vi "Experiment RT Servo.vi"(10 "Experiment Inputs":T2={"Duration"=5.0, "Initialisation Time"=1.0, "Sample Rate (Hz)"=200.0, "signal_type"=enum."Square", "Frequency"=0.5, "Amplitude"=1.0, "Offset"=2.5, "Velocity_feedback_gain"=0.1, "Feedforward_gain"=0.8, "LED_GAIN"=0.0, "LED_OFFSET"=0.0, "initial_condition"=0.0}) -> (0 "Error Out":errorcluster, 2 "Experiment Outputs":T4)   [LabVIEW 2016]
uses:
  Controls/Experiment Inputs.ctl
  Controls/Signal Type.ctl
  Controls/Experiment Outputs.ctl
  RT - Controls/Experiment RT State.ctl
  RT - Controls/Machine Data - RT.ctl
  <vilib>/Platform/TimedLoop/XDataNode/timing_clust.ctl
  <vilib>/Platform/TimedLoop/XDataNode/nitl_modes.ctl
  <vilib>/Platform/TimedLoop/XDataNode/wakeup.ctl
  Controller/Controller Values.ctl
  Pauseable Timer/Timer Mode.ctl
  <vilib>/Platform/TimedLoop/XDataNode/XDataNode.xnode
  <vilib>/ptbypt/NI_PtbyPt.lvlib
  <vilib>/Platform/TimedLoop/XDataNode/XDNodeRunTimeDep.lvlib
panel:
  out "Experiment RT State":T1
  in  "Error In":errorcluster
  out "Experiment Inputs Out":T2={"Duration"=5.0, "Initialisation Time"=1.0, "Sample Rate (Hz)"=200.0, "signal_type"=enum."Square", "Frequency"=0.5, "Amplitude"=1.0, "Offset"=2.5, "Velocity_feedback_gain"=0.1, "Feedforward_gain"=0.8, "LED_GAIN"=0.0, "LED_OFFSET"=0.0, "initial_condition"=0.0}
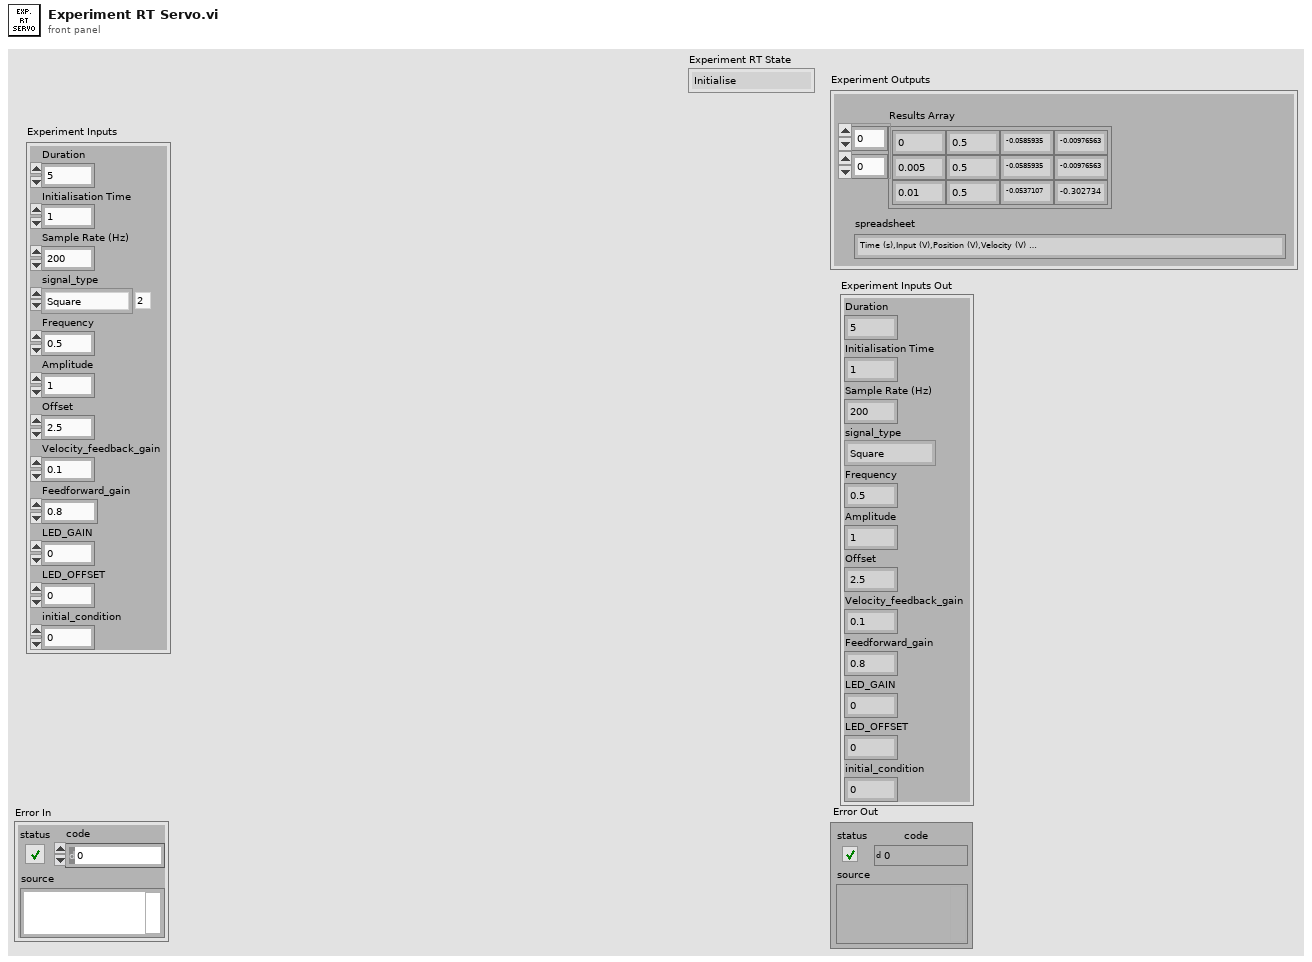
[diagram p1: front panel]
types:
  T1 = typedef "Experiment RT State.ctl" = enum16{"Initialise", "Wait Initialise", "Experiment", "End Experiment", "Quit"}
  T2 = typedef "Experiment Inputs.ctl" = cluster{"Duration":dbl, "Initialisation Time":dbl, "Sample Rate (Hz)":dbl, "signal_type":T3, "Frequency":dbl, "Amplitude":dbl, "Offset":dbl, "Velocity_feedback_gain":dbl, "Feedforward_gain":dbl, "LED_GAIN":dbl, "LED_OFFSET":dbl, "initial_condition":dbl}
  T3 = typedef "Signal Type.ctl" = enum16{"Sine", "Cosine", "Square", "Step"}
  T4 = typedef "Experiment Outputs.ctl" = cluster{"Results Array":dbl[][], "spreadsheet":string}
  T5 = typedef "Machine Data - RT.ctl" = cluster{"Results Array":dbl[][], "Motor Output":dbl, "LED Output":dbl, "Sample Index":u32, "Req. Samples":u32}
  T6 = typedef "XDNodeRunTimeDep.lvlib/timing_clust.ctl" = cluster{"Expected End [f-1]":u64, "Actual End [f-1]":u64, "Finished Late? [f-1]":bool, "Expected End [i-1]":u64, "Actual End [i-1]":u64, "Finished Late? [i-1]":bool, "Expected Start [i]":u64, "Actual Start [i]":u64, "Expected Start [f]":u64, "Actual Start [f]":u64, "Source Name":string, "Structure Name":string, "Period":i64, "Deadline":i64, "Offset":i64, "Start":i64, "Priority":i32, "Timeout":i32, "Mode":T7, "Wakeup Reason":T8, "Error":errorcluster, "Source Type":string, "Secondary Source Type":string, "Global End Time":u64, "Global Start Time":u64, "Frame Duration":u64, "Iteration Duration":u64, "Assigned CPU":i32, "I/O Scan Engine Mode":u32}
  T7 = typedef "XDNodeRunTimeDep.lvlib/nitl_modes.ctl" = enum32{"No Change", "Process missed periods, maintain original phase", "Discard missed periods, maintain original phase", "Process missed periods, ignore original phase", "Discard missed periods, ignore original phase"}
  T8 = typedef "XDNodeRunTimeDep.lvlib/wakeup.ctl" = enum32{"Normal", "Aborted", "Asynchronous wakeup", "Timing source error", "Timed loop error", "Timeout"}
  T9 = typedef "Controller Values.ctl" = cluster{"Ka":dbl, "Kt":dbl, "Offset":dbl}
  T10 = typedef "Timer Mode.ctl" = enum16{"Initialise", "Read", "Pause"}
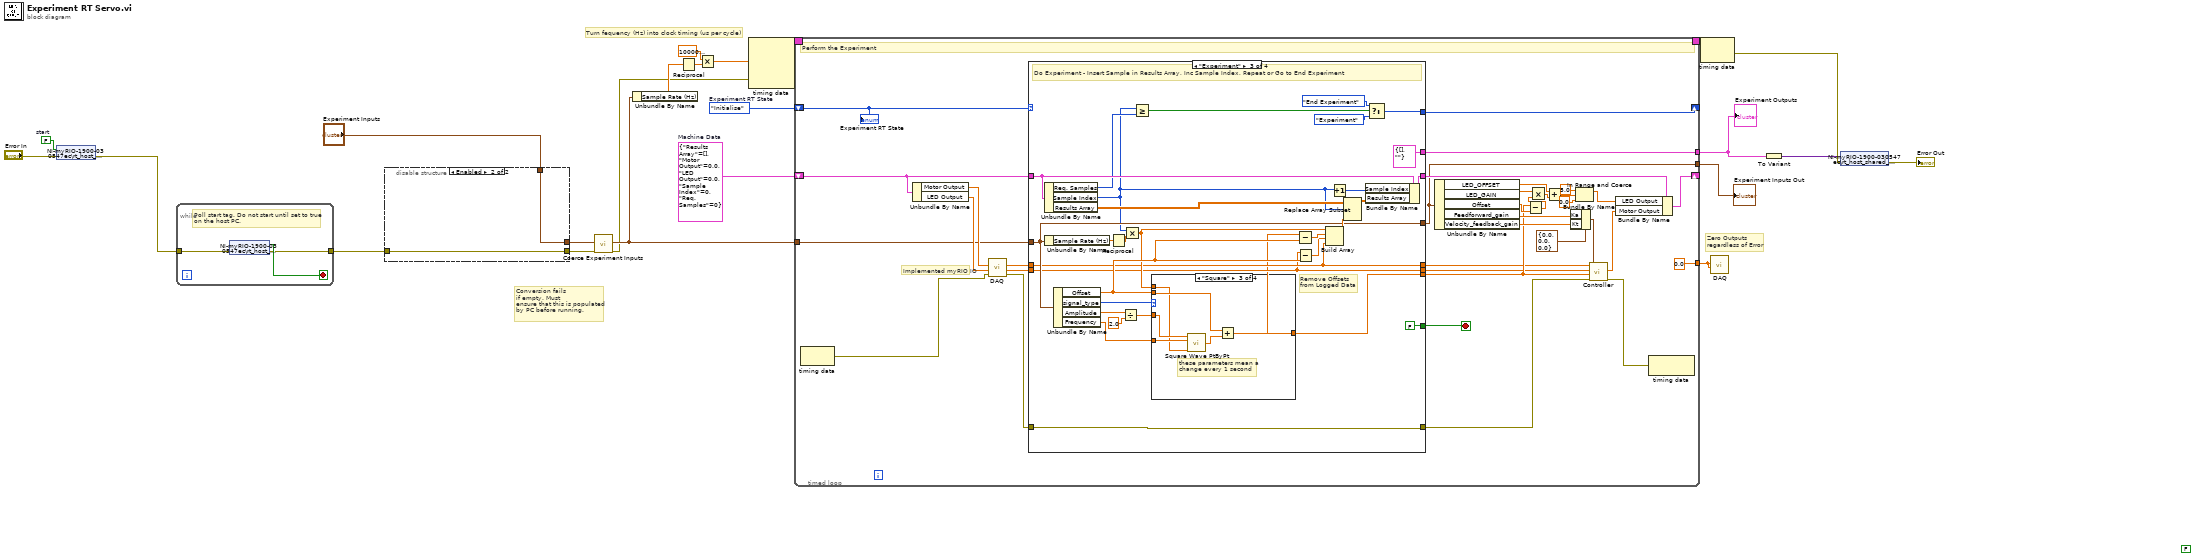
[diagram p0: block diagram]
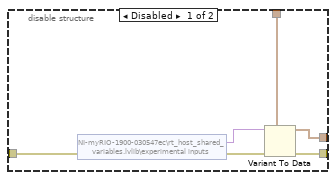
[diagram p2: hidden frame]
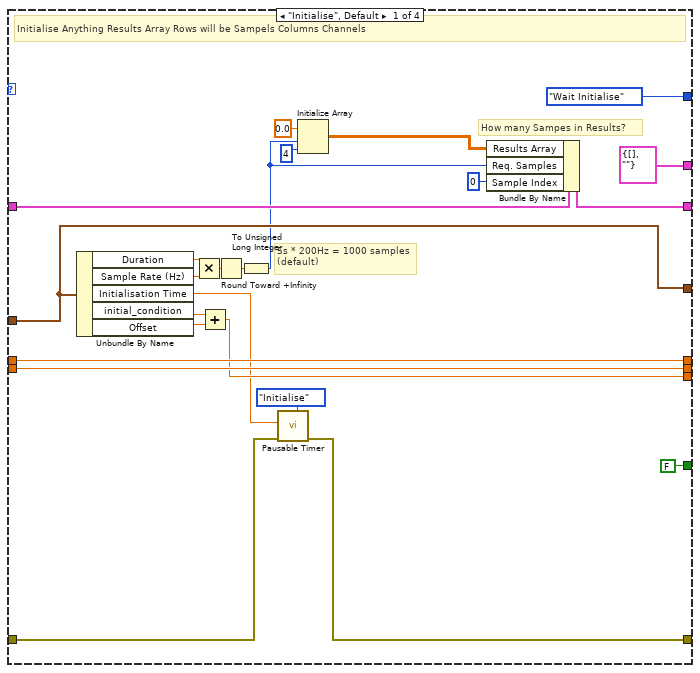
[diagram p3: hidden frame]
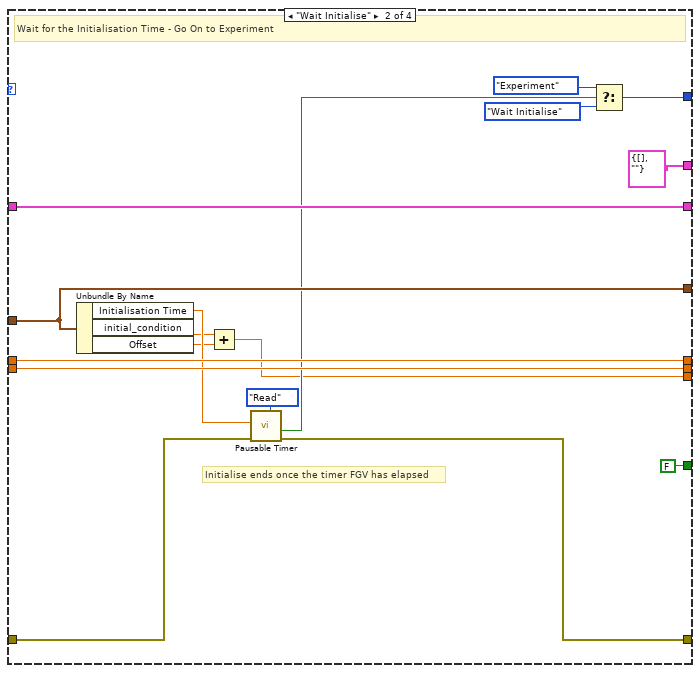
[diagram p4: hidden frame]
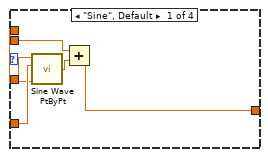
[diagram p5: hidden frame]
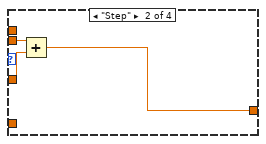
[diagram p6: hidden frame]
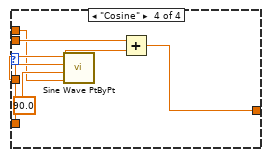
[diagram p7: hidden frame]
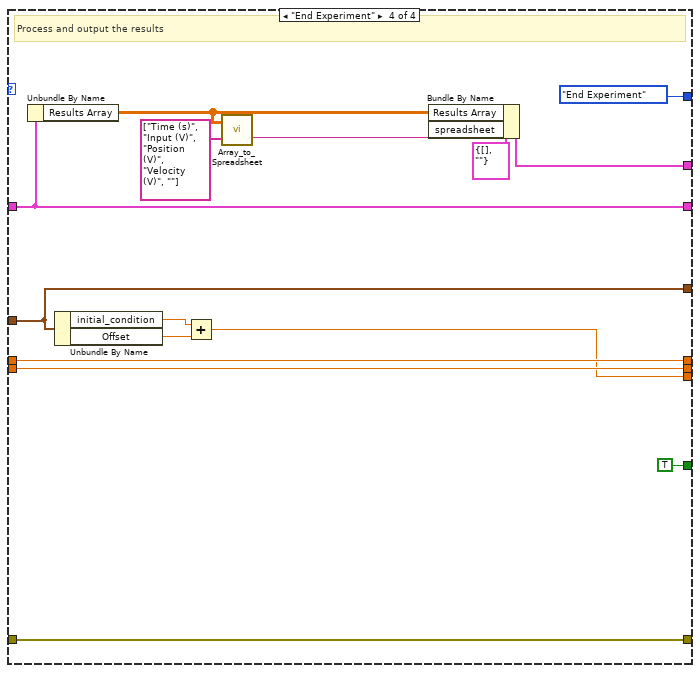
[diagram p8: hidden frame]
diagram:
  (unwired) FALSE
  w9 = T5 {"Results Array"=[], "Motor Output"=0.0, "LED Output"=0.0, "Sample Index"=0, "Req. Samples"=0}  # Machine Data
  w18 = Experiment_RT_State."Initialise"  # Experiment RT State
  w22 = FALSE  # start
  # "Conversion fails\nif empty. Must\nensure that this is populated\nby PC before running."
  # "Turn fequency (Hz) into clock timing (us per cycle)"
  # "Zero Outputs\nregardless of Error"
  n1 = shared-variable "NI-myRIO-1900-030547ec\\rt_host_shared_variables.lvlib\\start"(w22, error in="Error In") -> (error out=w21:errorcluster)
  n2 = while {
    tunnel: w21 -> [w25]
    tunnel: [w24] -> w5
    stop <- w26 stop-if-true
    # "Poll start tag. Do not start until set to true\non the host PC."
    n3 = shared-variable "NI-myRIO-1900-030547ec\\rt_host_shared_variables.lvlib\\start"(error in=w25) -> (w26:bool, error out=w24:errorcluster)
  }
  n4 = disable-structure shown="Enabled" {
    disable-tunnel: [w32 w34] -> w8
    disable-tunnel: "Experiment Inputs" -> [w31 w33]
    disable-tunnel: [w30 w33] -> w6
    disable-tunnel: w5 -> [w29 w34]
    frame Disabled {
      n5 = shared-variable "NI-myRIO-1900-030547ec\\rt_host_shared_variables.lvlib\\experimental inputs"(error in=w29) -> (w28:variant, error out=w27:errorcluster)
      n6 = Variant To Data(error in=w27, type=w31, Variant=w28) -> (data=w30:T2, error out=w32:errorcluster)
    }
    frame Enabled {
    }
  }
  n7 = call "Coerce Experiment Inputs.vi"("Error In"=w8, "Experiment Inputs"=w6) -> ("Error Out"=w10:errorcluster, "Experiment Inputs Out"=w17:T2)  [unwired: 8 in]
  n8 = Unbundle By Name(w17) -> ("Sample Rate (Hz)"=w16:dbl)
  n9 = Reciprocal(x=w16) -> (1/x=w15:dbl)
  n10 = Multiply(x=1000000.0 ("y"), y=w15) -> (x*y=w13:dbl)
  n11 = node-c288(w13, w10) -> (w20:T6)  [unwired: 2 in]
  n12 = timed-loop {
    shift-right: [w63] -> _
    shift-left: w18 -> [w64]
    shift-right: [w67] -> _
    shift-left: w9 -> [w68]
    timing: w20 -> [_]
    timing-out: [_] -> w19
    tunnel: w17 -> [w35]
    tunnel: [w62] -> w4
    tunnel: [0.0 ("Motor Output")] -> w12
    tunnel: [w49] -> w11
    stop <- w69 stop-if-true
    # "Implemented myRIO IO"
    # "Perform the Experiment"
    n13 = node-c288() -> (w65:errorcluster)  [unwired: 1 in]
    n14 = Unbundle By Name(w68) -> ("Motor Output"=w39:dbl, "LED Output"=w54:dbl)
    n15 = call "DAQ.vi"("Error In"=w65, "LED Output"=w54, "Motor Output"=w39) -> ("Error Out"=w56:errorcluster, "Position FB"=w40:dbl, "Tacho FB"=w41:dbl)  [unwired: 4 in, 2 out]
    n16 = case shown="\"Experiment\"" w64 {
      tunnel: [w90 w109 w123 w174] -> w61
      tunnel: w35 -> [w85 w108 w128 w172]
      tunnel: [FALSE FALSE FALSE TRUE] -> w69
      tunnel: w68 -> [w92 w104 w139 w171]
      tunnel: [w91 w104 w138 w171] -> w55
      tunnel: [w85 w108 w128 w172] -> w49
      tunnel: w56 -> [w83 w107 w123 w174]
      tunnel: [w84 w95 w111 w164] -> w42
      tunnel: w41 -> [w89 w106 w118 w176]
      tunnel: [w89 w106 w118 w176] -> w37
      tunnel: [w88 w105 w117 w175] -> w36
      tunnel: w40 -> [w88 w105 w117 w175]
      tunnel: [Experiment_RT_State."Wait Initialise" ("Experiment RT State") w103 w136 Experiment_RT_State."End Experiment" ("Experiment RT State")] -> w63
      tunnel: [T4 {"Results Array"=[], "spreadsheet"=""} ("Experiment Outputs") T4 {"Results Array"=[], "spreadsheet"=""} ("Experiment Outputs") T4 {"Results Array"=[], "spreadsheet"=""} ("Experiment Outputs") w167] -> w62
      frame "Initialise", Default {
        # "5s * 200Hz = 1000 samples\n(default)"
        # "How many Sampes in Results?"
        # "Initialise Anything Results Array Rows will be Sampels Columns Channels"
        n17 = Unbundle By Name(w85) -> ("Duration"=w81:dbl, "Sample Rate (Hz)"=w80:dbl, "Initialisation Time"=w82:dbl, "initial_condition"=w72:dbl, "Offset"=w71:dbl)
        n18 = Multiply(x=w81, y=w80) -> (x*y=w79:dbl)
        n19 = Add(x=w72, y=w71) -> (x+y=w84:dbl)
        n20 = Round Toward +Infinity(x=w79) -> (ceil(x): smallest int >= x=w78:dbl)
        n21 = To Unsigned Long Integer(number=w78) -> (unsigned 32bit integer=w73:u32)
        n22 = call "Pausable Timer.vi"("Timer Mode"=Timer_Mode."Initialise", "Error In"=w83, "Desired Time (S)"=w82) -> ("Error Out"=w90:errorcluster)  [unwired: 6 in, 2 out]
        n23 = Initialize Array(0.0 ("element"), w73, 4 ("dimension size")) -> (w75:dbl[][])
        n24 = Bundle By Name(cluster=w92, "Results Array"=w75, "Req. Samples"=w73, "Sample Index"=u32 0) -> (w91:T5)
      }
      frame "Wait Initialise" {
        # "Initialise ends once the timer FGV has elapsed"
        # "Wait for the Initialisation Time - Go On to Experiment"
        n25 = Unbundle By Name(w108) -> ("Initialisation Time"=w101:dbl, "initial_condition"=w96:dbl, "Offset"=w94:dbl)
        n26 = Add(x=w96, y=w94) -> (x+y=w95:dbl)
        n27 = call "Pausable Timer.vi"("Timer Mode"=Timer_Mode."Read", "Error In"=w107, "Desired Time (S)"=w101) -> ("Error Out"=w109:errorcluster, "Time Up?"=w100:bool)  [unwired: 6 in, 1 out]
        n28 = Select(t=Experiment_RT_State."Experiment" ("Experiment RT State"), s=w100, f=Experiment_RT_State."Wait Initialise" ("Experiment RT State")) -> (s? t:f=w103:T1)
      }
      frame "Experiment" {
        # "Remove Offsets\nfrom Logged Data"
        # "Do Experiment - Insert Sample in Results Array, Inc Sample Index, Repeat or Go to End Experiment"
        n29 = Unbundle By Name(w139) -> ("Req. Samples"=w132:u32, "Sample Index"=w127:u32, "Results Array"=w130:dbl[][])
        n30 = Unbundle By Name(w128) -> ("Sample Rate (Hz)"=w125:dbl)
        n31 = Unbundle By Name(w128) -> ("Offset"=w120:dbl, "signal_type"=w122:T3, "Amplitude"=w113:dbl, "Frequency"=w121:dbl)
        n32 = Reciprocal(x=w125) -> (1/x=w124:dbl)
        n33 = Divide(x=w113, y=2.0) -> (x/y=w114:dbl)
        n34 = Multiply(x=w127, y=w124) -> (x*y=w119:dbl)
        n35 = Greater Or Equal?(x=w127, y=w132) -> (x >= y?=w133:bool)
        n36 = case shown="\"Square\"" w122 {
          tunnel: w114 -> [w146 w148 w155 w161]
          tunnel: w121 -> [w145 _ w154 w160]
          tunnel: w120 -> [w143 w149 w152 w157]
          tunnel: [w142 w147 w150 w158] -> w111
          tunnel: w119 -> [w141 _ w151 w156]
          frame "Sine", Default {
            n37 = call <vilib>:"Sine Wave PtByPt.vi"("time"=w141, "frequency"=w145, "amplitude"=w146) -> ("sine wave"=w144:dbl)  [unwired: 1 in]
            n38 = Add(x=w143, y=w144) -> (x+y=w142:dbl)
          }
          frame "Step" {
            n39 = Add(x=w149, y=w148) -> (x+y=w147:dbl)
          }
          frame "Square" {
            # "these parameters mean a\nchange every 1 second"
            n40 = call <vilib>:"Square Wave PtByPt.vi"("amplitude"=w155, "frequency"=w154, "time"=w151) -> ("square wave"=w153:dbl)  [unwired: 2 in]
            n41 = Add(x=w152, y=w153) -> (x+y=w150:dbl)
          }
          frame "Cosine" {
            n42 = call <vilib>:"Sine Wave PtByPt.vi"("time"=w156, "phase"=90.0, "frequency"=w160, "amplitude"=w161) -> ("sine wave"=w159:dbl)
            n43 = Add(x=w157, y=w159) -> (x+y=w158:dbl)
          }
        }
        n44 = Subtract(x=w111, y=w120) -> (x-y=w116:dbl)
        n45 = Subtract(x=w117, y=w120) -> (x-y=w115:dbl)
        n46 = Build Array(w119, w116, w115, w118) -> (w129:dbl[])
        n47 = Increment(x=w127) -> (x+1=w137:u32)
        n48 = Replace Array Subset(array=w130, new element=w129, index (row)=w127) -> (w131:dbl[][])  [unwired: 1 in]
        n49 = Bundle By Name(cluster=w139, "Sample Index"=w137, "Results Array"=w131) -> (w138:T5)
        n50 = Select(t=Experiment_RT_State."End Experiment" ("Experiment RT State"), s=w133, f=Experiment_RT_State."Experiment" ("Experiment RT State")) -> (s? t:f=w136:T1)
      }
      frame "End Experiment" {
        # "Process and output the results"
        n51 = Unbundle By Name(w171) -> ("Results Array"=w163:dbl[][])
        n52 = Unbundle By Name(w172) -> ("initial_condition"=w165:dbl, "Offset"=w166:dbl)
        n53 = Add(x=w165, y=w166) -> (x+y=w164:dbl)
        n54 = call "Array_to_Spreadsheet.vi"("Headers"=string[] ["Time (s)", "Input (V)", "Position (V)", "Velocity (V)", ""], "Input Array"=w163) -> ("spreadsheet string"=w170:string)
        n55 = Bundle By Name(cluster=T4 {"Results Array"=[], "spreadsheet"=""} ("Experiment Outputs"), "Results Array"=w163, "spreadsheet"=w170) -> (w167:T4)
      }
    }
    n56 = Unbundle By Name(w49) -> ("LED_OFFSET"=w51:dbl, "LED_GAIN"=w53:dbl, "Offset"=w47:dbl, "Feedforward_gain"=w58:dbl, "Velocity_feedback_gain"=w57:dbl)
    n57 = Subtract(x=w42, y=w47) -> (x-y=w48:dbl)
    n58 = Multiply(x=w53, y=w48) -> (x*y=w52:dbl)
    n59 = Add(x=w51, y=w52) -> (x+y=w46:dbl)
    n60 = Bundle By Name(cluster=T9 {"Ka"=0.0, "Kt"=0.0, "Offset"=0.0} ("Controller Values"), "Ka"=w58, "Kt"=w57) -> (w59:T9)
    n61 = In Range and Coerce(upper limit=5.0, x=w46, lower limit=0.0) -> (coerced(x)=w43:dbl)  [unwired: 1 out]
    n62 = call "Controller.vi"("Controller Values"=w59, "Error In"=w61, "Set Point"=w42, "Position FB"=w36, "Tacho FB"=w37) -> ("Error Out"=w66:errorcluster, "Controller Out"=w38:dbl)  [unwired: 5 in]
    n63 = Bundle By Name(cluster=w55, "LED Output"=w43, "Motor Output"=w38) -> (w67:T5)
    n64 = node-c288(w66) -> ()  [unwired: 1 out]
    "Experiment RT State" <- w64
  }
  "Experiment Outputs" <- w4
  "Experiment Inputs Out" <- w11
  n65 = node-c288(w19) -> (w3:errorcluster)
  n66 = call "DAQ.vi"("LED Output"=w12, "Motor Output"=w12) -> ()  [unwired: 5 in, 5 out]
  n67 = To Variant(anything=w4) -> (Variant=w2:variant)
  n68 = shared-variable "NI-myRIO-1900-030547ec\\rt_host_shared_variables.lvlib\\Output"(w2, error in=w3) -> (error out=→"Error Out":errorcluster)
